vi "Init.vi"(8 "error in (no error)":errorcluster, 10 "Intrs Configs":T1, 11 "MSS Actor in":refnum<class "MSS Remote Actor.lvclass">) -> (0 "error out":errorcluster, 3 "MSS Actor out":refnum<class "MSS Remote Actor.lvclass">)   [LabVIEW 2023, in "MSS Remote Actor.lvlib" / "MSS Remote Actor.lvclass"]
uses:
  MSS Remote Actor.lvclass
  MSS Remote Actor.lvclass/MSS Remote Actor.ctl
  HAL GOOP4/Measure and Stimulus Subsystems/Measure and Stimulus Subsystems.lvclass
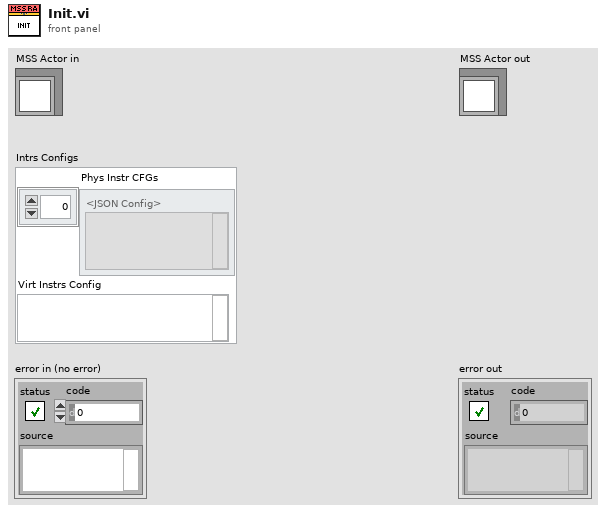
[diagram p1: front panel]
types:
  T1 = cluster{"Phys Instr CFGs":string[], "Virt Instrs Config":string}
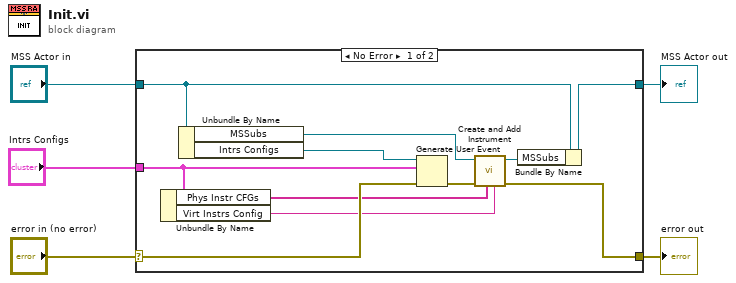
[diagram p0: block diagram]
diagram:
  n1 = case shown="No Error" "error in (no error)" {
    selector: "error in (no error)" -> [w15 w17]
    tunnel: [w11 w17] -> w4
    tunnel: [w8 w18] -> w2
    tunnel: "MSS Actor in" -> [w14 w18]
    tunnel: "Intrs Configs" -> [w6 _]
    frame No Error {
      n2 = Unbundle By Name(w6) -> ("Phys Instr CFGs"=w10:string[], "Virt Instrs Config"=w9:string)
      n3 = Unbundle By Name(w14) -> ("MSSubs"=w13:refnum<class "Measure and Stimulus Subsystems.lvclass">, "Intrs Configs"=w16:refnum<user-event>)
      n4 = Generate User Event(user event=w16, event data cluster=w6, error in=w15) -> (error out=w12:errorcluster)  [unwired: 1 in, 1 out]
      n5 = call-dynamic "Create and Add Instrument.vi"("Virt Instr JSON Config"=w9, "Physical Intr Configs"=w10, "Error In"=w12, "reference in"=w13) -> ("Error Out"=w11:errorcluster, "reference out"=w7:refnum<class "Measure and Stimulus Subsystems.lvclass">)  [unwired: 6 in]
      n6 = Bundle By Name(cluster=w14, "MSSubs"=w7) -> (w8:refnum<class "MSS Remote Actor.lvclass">)
    }
    frame Error {
    }
  }
  "error out" <- w4
  "MSS Actor out" <- w2
